vi "流水灯.vi"() -> ()   [LabVIEW 2017]
panel:
  in  "毫秒":i32=100
  in  "正？":bool
  in  "反转":bool
  out "簇":T1
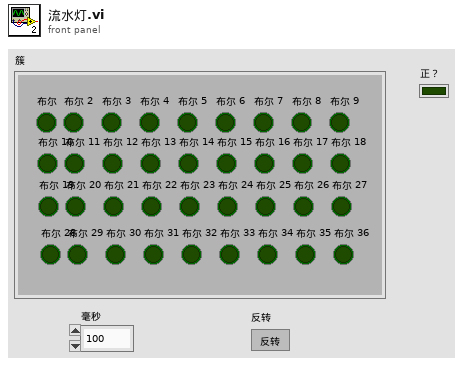
[diagram p1: front panel]
types:
  T1 = cluster{"布尔":bool, "布尔 2":bool, "布尔 3":bool, "布尔 4":bool, "布尔 5":bool, "布尔 6":bool, "布尔 7":bool, "布尔 8":bool, "布尔 9":bool, "布尔 10":bool, "布尔 11":bool, "布尔 12":bool, "布尔 13":bool, "布尔 14":bool, "布尔 15":bool, "布尔 16":bool, "布尔 17":bool, "布尔 18":bool, "布尔 19":bool, "布尔 20":bool, "布尔 21":bool, "布尔 22":bool, "布尔 23":bool, "布尔 24":bool, "布尔 25":bool, "布尔 26":bool, "布尔 27":bool, "布尔 28":bool, "布尔 29":bool, "布尔 30":bool, "布尔 31":bool, "布尔 32":bool, "布尔 33":bool, "布尔 34":bool, "布尔 35":bool, "布尔 36":bool}
  T2 = cluster{"[0]":bool, "[1]":bool, "[2]":bool, "[3]":bool, "[4]":bool, "[5]":bool, "[6]":bool, "[7]":bool, "[8]":bool, "[9]":bool, "[10]":bool, "[11]":bool, "[12]":bool, "[13]":bool, "[14]":bool, "[15]":bool, "[16]":bool, "[17]":bool, "[18]":bool, "[19]":bool, "[20]":bool, "[21]":bool, "[22]":bool, "[23]":bool, "[24]":bool, "[25]":bool, "[26]":bool, "[27]":bool, "[28]":bool, "[29]":bool, "[30]":bool, "[31]":bool, "[32]":bool, "[33]":bool, "[34]":bool, "[35]":bool}
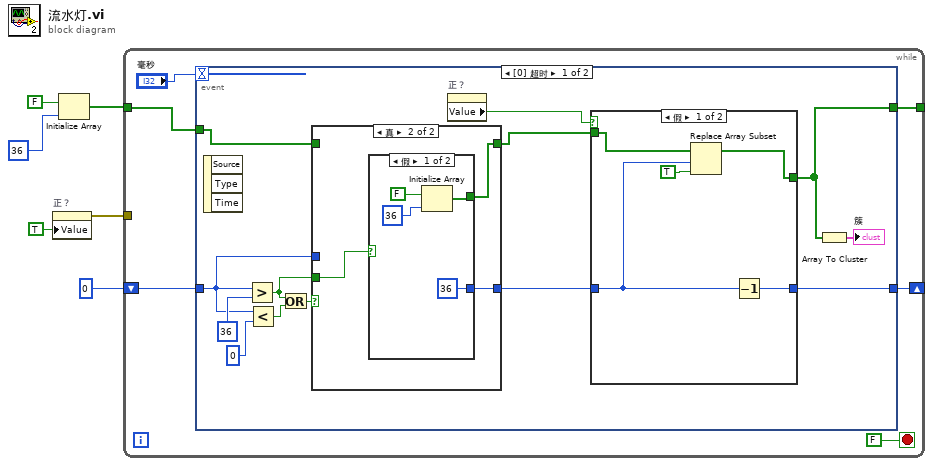
[diagram p0: block diagram]
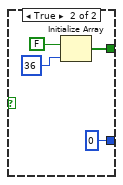
[diagram p3: hidden frame]
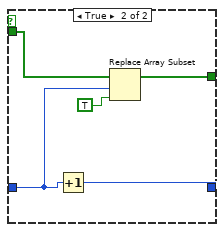
[diagram p4: hidden frame]
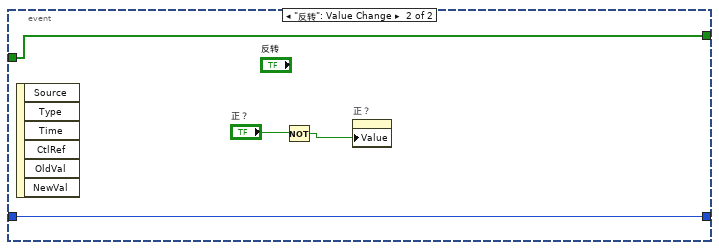
[diagram p5: hidden frame]
diagram:
  n1 = property on="正？" class="Bool (严格)"("Value"=TRUE ("正？")) -> (error out=w1:errorcluster)  [unwired: 2 in, 1 out]
  n2 = Initialize Array(FALSE, 36 ("维数大小")) -> (w4:bool[])
  n3 = while {
    shift-right: [w8] -> _
    shift-left: 0 -> [w10]
    tunnel: w1 -> [_]
    tunnel: w4 -> [w11]
    tunnel: [w9] -> _
    stop <- FALSE stop-if-true
    n4 = event shown="[0] 超时" {
      selector: _ -> [_ _]
      dyn-events: _ -> [_ _]
      timeout: "毫秒" -> [_ _]
      tunnel: w11 -> [w19 w52]
      tunnel: w10 -> [w17 w51]
      tunnel: [w24 w52] -> w9
      tunnel: [w22 w51] -> w8
      event Timeout {
        n5 = event-data() -> ()  [unwired: 1 in, 3 out]
        n6 = Greater?(x=w17, y=36) -> (0:w13:bool)
        n7 = Less?(x=w17, y=0) -> (x < y?=w15:bool)
        n8 = Or(x=w13, y=w15) -> (x .or. y?=w14:bool)
        n9 = case shown="真" w14 {
          tunnel: [w27 w30] -> w20
          tunnel: w17 -> [w27 _]
          tunnel: w19 -> [w26 _]
          tunnel: [w26 w29] -> w18
          tunnel: w13 -> [_ w28]
          frame False {
          }
          frame True {
            n10 = case shown="假" w28 {
              tunnel: [36 0] -> w30
              tunnel: [w32 w35] -> w29
              frame False {
                n11 = Initialize Array(FALSE, 36 ("维数大小")) -> (w32:bool[])
              }
              frame True {
                n12 = Initialize Array(FALSE, 36 ("维数大小")) -> (w35:bool[])
              }
            }
          }
        }
        n13 = property on="正？" class="Bool (严格)"() -> ("Value"=w25:bool)  [unwired: 2 in, 2 out]
        n14 = case shown="假" w25 {
          tunnel: w18 -> [w42 w48]
          tunnel: w20 -> [w39 w45]
          tunnel: [w40 w46] -> w24
          tunnel: [w41 w44] -> w22
          frame False {
            n15 = Replace Array Subset(array=w42, new element=TRUE ("新元素/子数组"), index=w39) -> (w40:bool[])
            n16 = Decrement(x=w39) -> (x-1=w41:i32)
          }
          frame True {
            n17 = Increment(x=w45) -> (x+1=w44:i32)
            n18 = Replace Array Subset(array=w48, new element=TRUE ("新元素/子数组"), index=w45) -> (w46:bool[])
          }
        }
        n19 = Array To Cluster(array=w24) -> (cluster=→"簇":T2)
      }
      event "反转": Value Change {
        n20 = event-data() -> ()  [unwired: 1 in, 6 out]
        n21 = Not(x="正？") -> (.not. x?=w49:bool)
        n22 = property on="正？" class="Bool (严格)"("Value"=w49) -> ()  [unwired: 2 in, 2 out]
      }
    }
  }
